vi "Filter Packets Persona.vi"(10 "Boolean":bool, 11 "LiveData in":T1 {"Reference/Temperature 2" format="%.2f"; "Accelerometer" format="%.2f"; "Battery" format="%.2f"; "Reference/Temperature 1" format="%.2f"; "LoadSensors" format="%.2f"}) -> (3 "LiveData out":T1 {"Reference/Temperature 2" format="%.2f"; "Accelerometer" format="%.2f"; "Battery" format="%.2f"; "Reference/Temperature 1" format="%.2f"; "LoadSensors" format="%.2f"})   [LabVIEW 2015]
uses:
  Controls/LiveData.ctl
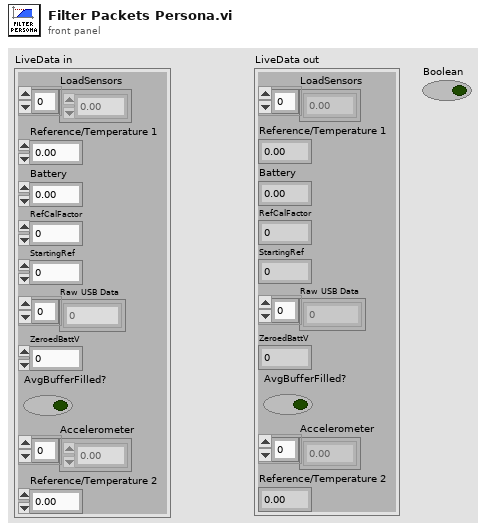
[diagram p1: front panel]
types:
  T1 = typedef "LiveData.ctl" = cluster{"LoadSensors":dbl[], "Reference/Temperature 1":dbl, "Battery":dbl, "RefCalFactor":dbl, "StartingRef":dbl, "Raw USB Data":u16[], "ZeroedBattV":dbl, "AvgBufferFilled?":bool, "Accelerometer":dbl[], "Reference/Temperature 2":dbl}
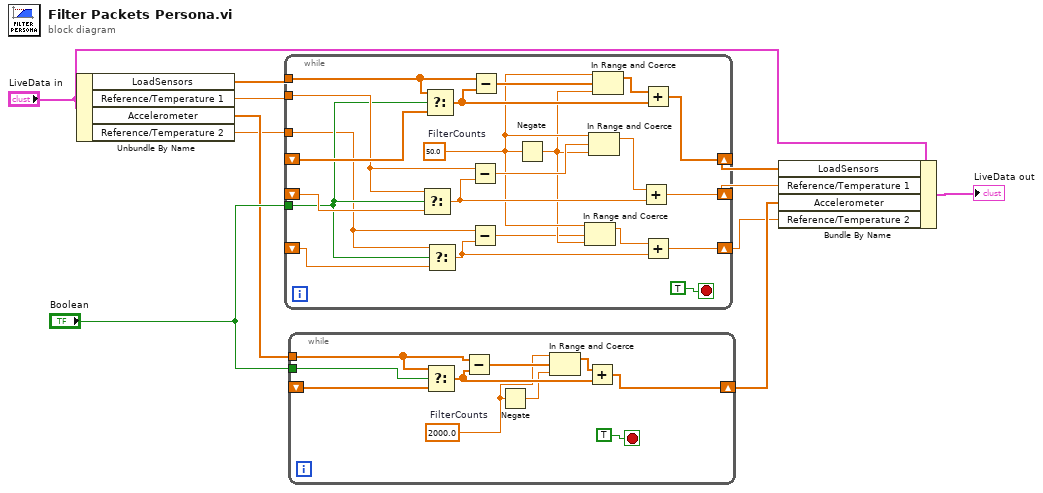
[diagram p0: block diagram]
diagram:
  n1 = Unbundle By Name("LiveData in") -> ("LoadSensors"=w4:dbl[], "Reference/Temperature 1"=w5:dbl, "Accelerometer"=w9:dbl[], "Reference/Temperature 2"=w2:dbl)
  n2 = while {
    shift-right: [w18] -> w7
    shift-left: _ -> [w30]
    tunnel: w4 -> [w29]
    shift-right: [w28] -> w8
    shift-left: _ -> [w26]
    tunnel: w5 -> [w27]
    tunnel: "Boolean" -> [w21]
    tunnel: w2 -> [w20]
    shift-right: [w13] -> w1
    shift-left: _ -> [w12]
    stop <- TRUE stop-if-true
    w19 = 50.0  # FilterCounts
    n3 = Select(t=w27, s=w21, f=w26) -> (s? t:f=w25:dbl)
    n4 = Select(t=w29, s=w21, f=w30) -> (s? t:f=w31:dbl[])
    n5 = Select(t=w20, s=w21, f=w12) -> (s? t:f=w14:dbl)
    n6 = Subtract(x=w27, y=w25) -> (x-y=w23:dbl)
    n7 = Subtract(x=w20, y=w14) -> (x-y=w15:dbl)
    n8 = Subtract(x=w29, y=w31) -> (x-y=w33:dbl[])
    n9 = Negate(x=w19) -> (-x=w17:dbl)
    n10 = In Range and Coerce(upper limit=w19, x=w15, lower limit=w17) -> (coerced(x)=w16:dbl)  [unwired: 1 out]
    n11 = In Range and Coerce(upper limit=w19, x=w23, lower limit=w17) -> (coerced(x)=w24:dbl)  [unwired: 1 out]
    n12 = In Range and Coerce(upper limit=w19, x=w33, lower limit=w17) -> (coerced(x)=w32:dbl[])  [unwired: 1 out]
    n13 = Add(x=w24, y=w25) -> (x+y=w28:dbl)
    n14 = Add(x=w32, y=w31) -> (x+y=w18:dbl[])
    n15 = Add(x=w16, y=w14) -> (x+y=w13:dbl)
  }
  n16 = while {
    shift-right: [w39] -> w11
    shift-left: _ -> [w40]
    tunnel: "Boolean" -> [w37]
    tunnel: w9 -> [w34]
    stop <- TRUE stop-if-true
    w35 = 2000.0  # FilterCounts
    n17 = Select(t=w34, s=w37, f=w40) -> (s? t:f=w41:dbl[])
    n18 = Subtract(x=w34, y=w41) -> (x-y=w43:dbl[])
    n19 = Negate(x=w35) -> (-x=w36:dbl)
    n20 = In Range and Coerce(upper limit=w35, x=w43, lower limit=w36) -> (coerced(x)=w42:dbl[])  [unwired: 1 out]
    n21 = Add(x=w42, y=w41) -> (x+y=w39:dbl[])
  }
  n22 = Bundle By Name(cluster="LiveData in", "LoadSensors"=w7, "Reference/Temperature 1"=w8, "Accelerometer"=w11, "Reference/Temperature 2"=w1) -> (→"LiveData out":T1)
